vi "Find Virtual Sensor Readings NIARC 2016 Course (SubVI).vi"(8 "Lidar's Maximum Viewing Distance":dbl=5.6, 9 "Lidar Viewing Angle (degrees)":dbl=240.0, 10 "Number of Lidar Measurements":dbl=683.0, 11 "Position":cluster{"X":dbl, "Y":dbl, "Angle":dbl}) -> (1 "Angle":dbl[](array[numeric]), 2 "Magnitude":dbl[](array[numeric]))   [LabVIEW 2015]
panel:
  out "Polar Plot":picture
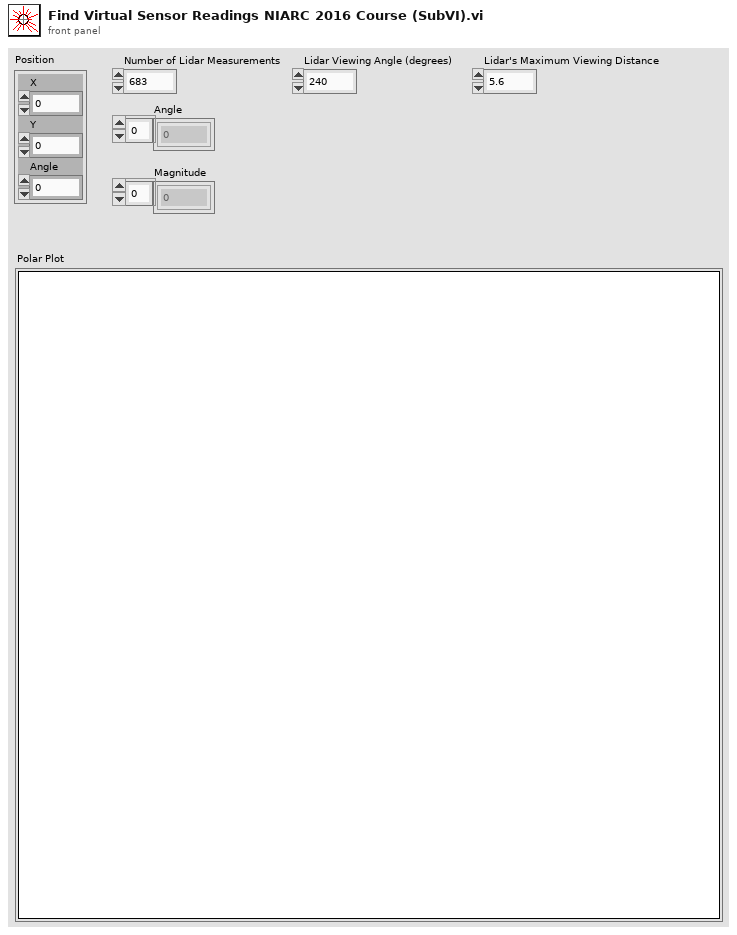
[diagram p1: front panel]
types:
  T1 = typedef "LVBoundsTypeDef.ctl" = cluster{"Width":u32, "Height":u32}
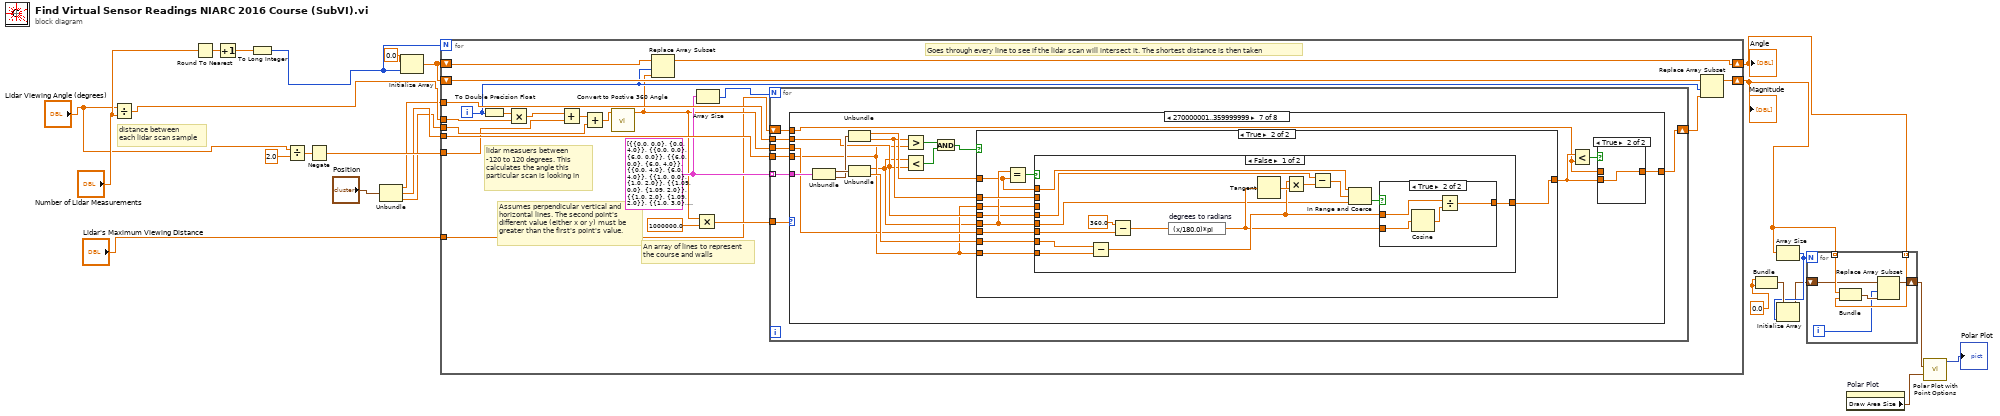
[diagram p0: block diagram]
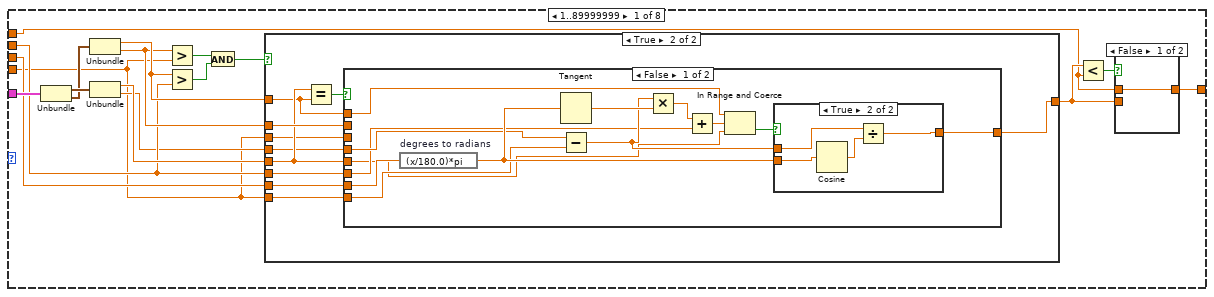
[diagram p2: hidden frame]
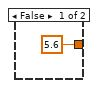
[diagram p4: hidden frame]
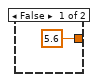
[diagram p5: hidden frame]
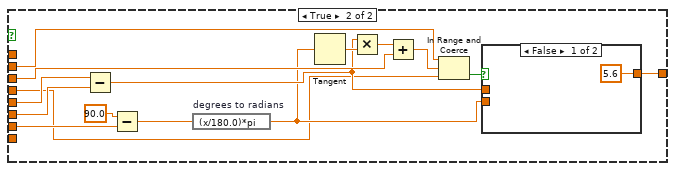
[diagram p6: hidden frame]
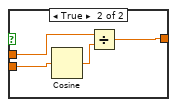
[diagram p7: hidden frame]
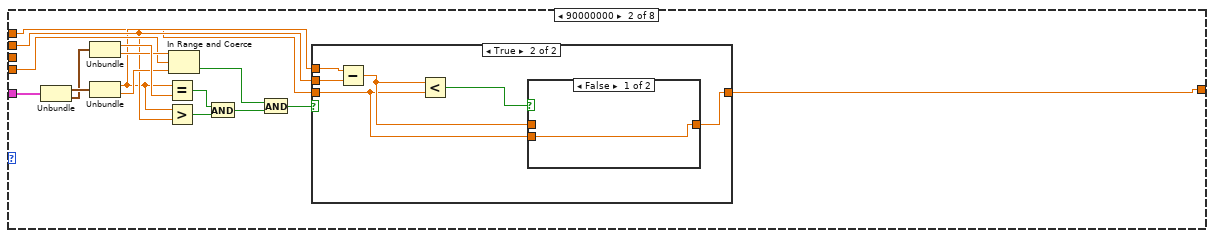
[diagram p8: hidden frame]
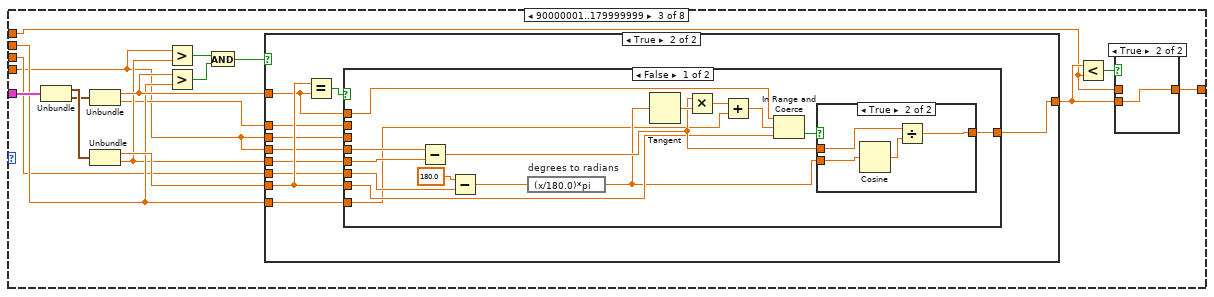
[diagram p11: hidden frame]
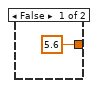
[diagram p13: hidden frame]
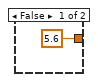
[diagram p14: hidden frame]
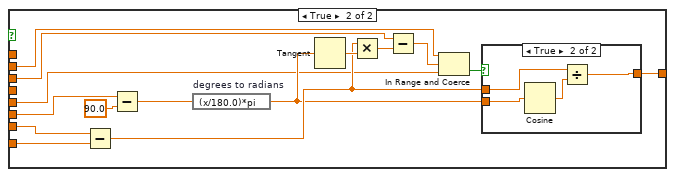
[diagram p15: hidden frame]
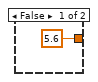
[diagram p16: hidden frame]
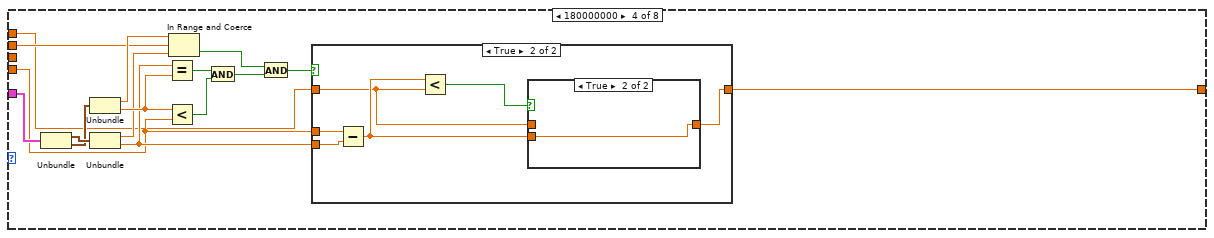
[diagram p17: hidden frame]
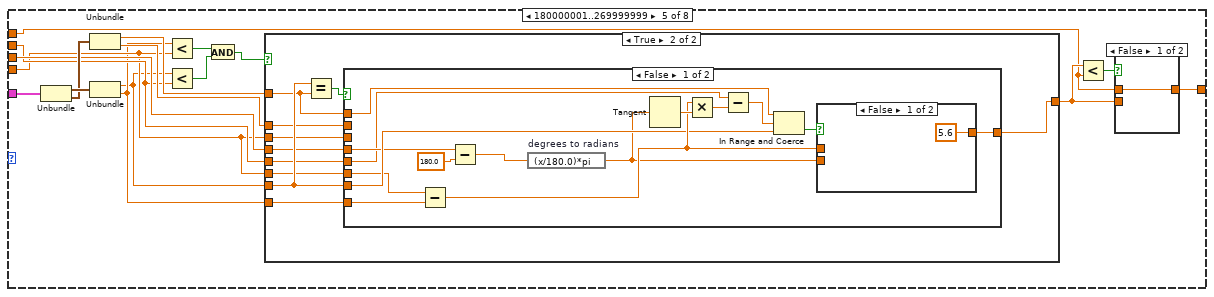
[diagram p20: hidden frame]
diagram:
  w4 = 0.0
  # "distance between\neach lidar scan sample"
  n1 = Divide(x="Lidar Viewing Angle (degrees)", y="Number of Lidar Measurements") -> (x/y=w22:dbl)
  n2 = Round To Nearest(number="Number of Lidar Measurements") -> (nearest integer value=w25:dbl)
  n3 = Increment(x=w25) -> (x+1=w24:dbl)
  n4 = To Long Integer(number=w24) -> (32bit integer=w23:i32)
  n5 = Divide(x="Lidar Viewing Angle (degrees)", y=2.0) -> (x/y=w19:dbl)
  n6 = Negate(x=w19) -> (-x=w16:dbl)
  n7 = Unbundle("Position") -> ("X"=w12:dbl, "Y"=w11:dbl, "Angle"=w10:dbl)
  n8 = Initialize Array(0.0 ("element"), w23) -> (w14:dbl[])
  n9 = for {
    N: w23 -> [_]
    tunnel: w10 -> [w40]
    tunnel: w12 -> [w45]
    tunnel: w11 -> [w44]
    tunnel: w22 -> [w43]
    shift-right: [w36] -> w7
    shift-left: w14 -> [w37]
    shift-right: [w28] -> w6
    shift-left: w14 -> [w30]
    tunnel: "Lidar's Maximum Viewing Distance" -> [w27]
    tunnel: w16 -> [w26]
    i -> [w31]
    w35 = cluster{cluster{dbl, dbl}, cluster{dbl, dbl}}[] [{{0.0, 0.0}, {0.0, 4.0}}, {{0.0, 0.0}, {6.0, 0.0}}, {{6.0, 0.0}, {6.0, 4.0}}, {{0.0, 4.0}, {6.0, 4.0}}, {{1.0, 0.0}, {1.0, 2.0}}, {{1.09, 0.0}, {1.09, 2.0}}, {{1.0, 2.0}, {1.09, 2.0}}, {{1.0, 3.0}, {1.0, 4.0}}, {{1.09, 3.0}, {1.09, 4.0}}, {{1.0, 3.0}, {1.09, 3.0}}, {{1.5, 3.88}, {1.5, 4.0}}, {{4.0, 3.88}, {4.0, 4.0}}, {{1.5, 3.88}, {4.0, 3.88}}, {{1.25, 0.0}, {1.25, 0.12}}, {{2.25, 0.0}, {2.25, 0.12}}, {{1.25, 0.12}, {2.25, 0.12}}, {{3.5, 0.0}, {3.5, 2.09}}, {{3.59, 0.0}, {3.59, 2.0}}, {{3.5, 2.09}, {4.5, 2.09}}, {{4.5, 2.0}, {4.5, 2.09}}, {{3.59, 2.0}, {4.5, 2.0}}, {{3.8, 0.0}, {3.8, 0.12}}, {{5.8, 0.0}, {5.8, 0.12}}, {{3.8, 0.12}, {5.8, 0.12}}]
    # "Assumes perpendicular vertical and\nhorizontal lines. The second point's\ndifferent value (either x or y) must be\ngreater than the first's point's value."
    # "Goes through every line to see if the lidar scan will intersect it. The shortest distance is then taken"
    # "An array of lines to represent\nthe course and walls"
    # "lidar measuers between\n-120 to 120 degrees. This\ncalculates the angle this \nparticular scan is looking in"
    n10 = To Double Precision Float(number=w31) -> (double precision float=w42:dbl)
    n11 = Multiply(x=w42, y=w43) -> (x*y=w41:dbl)
    n12 = Add(x=w41, y=w26) -> (x+y=w39:dbl)
    n13 = Add(x=w39, y=w40) -> (x+y=w32:dbl)
    n14 = call "Convert to Postive 360 Angle.vi"("Angle in"=w32) -> ("Angle out"=w29:dbl)  [unwired: 10 in]
    n15 = Replace Array Subset(array=w30, new element=w29, index=w31) -> (w28:dbl[])
    n16 = Multiply(x=w29, y=1000000.0) -> (x*y=w33:dbl)
    n17 = Array Size(array=w35) -> (size(s)=w46:i32)
    n18 = for {
      N: w46 -> [_]
      tunnel: w35 -> [w53] mode=indexing
      tunnel: w44 -> [w52]
      tunnel: w45 -> [w51]
      shift-right: [w49] -> w38
      shift-left: w27 -> [w50]
      tunnel: w29 -> [w48]
      tunnel: w33 -> [w47]
      n19 = case shown="270000001..359999999" w47 {
        tunnel: w53 -> [w68 w130 w155 w221 w249 w316 w343 w422]
        tunnel: w52 -> [w54 w126 w147 w220 w245 w313 w339 w409]
        tunnel: w51 -> [w61 w125 w153 w219 w247 w312 w340 w416]
        tunnel: w50 -> [w56 w123 w148 w218 w246 w314 w341 w408]
        tunnel: [w58 w122 w149 w217 w242 w315 w338 w407] -> w49
        tunnel: w48 -> [w60 _ w152 _ w248 _ w342 _]
        frame 1..89999999 {
          n20 = Unbundle(w68) -> (w70:cluster{dbl, dbl}, w69:cluster{dbl, dbl})
          n21 = Unbundle(w69) -> (w63:dbl, w62:dbl)
          n22 = Unbundle(w70) -> (w64:dbl, w55:dbl)
          n23 = Greater?(x=w62, y=w54) -> (0:w67:bool)
          n24 = Greater?(x=w63, y=w61) -> (0:w66:bool)
          n25 = And(x=w67, y=w66) -> (x .and. y?=w65:bool)
          n26 = case shown="True" w65 {
            tunnel: [5.6 w77] -> w57
            tunnel: w64 -> [_ w81]
            tunnel: w63 -> [_ w74]
            tunnel: w62 -> [_ w82]
            tunnel: w61 -> [_ w80]
            tunnel: w60 -> [_ w79]
            tunnel: w54 -> [_ w78]
            tunnel: w55 -> [_ w76]
            tunnel: w54 -> [_ w75]
            frame False {
            }
            frame True {
              n27 = Equal?(x=w81, y=w74) -> (x = y?=w83:bool)
              n28 = case shown="False" w83 {
                tunnel: w82 -> [_ w105]
                tunnel: w81 -> [w84 w116]
                tunnel: w80 -> [w89 w115]
                tunnel: w79 -> [w90 w114]
                tunnel: w78 -> [_ w109]
                tunnel: [w88 w106] -> w77
                tunnel: w76 -> [w92 w104]
                tunnel: w75 -> [w91 _]
                tunnel: w74 -> [w87 _]
                frame False {
                  n29 = expression code="(x/180.0)*pi" "degrees to radians"(w90) -> (w93:dbl)
                  n30 = Tangent(1:w93) -> (0:w96:dbl)
                  n31 = Subtract(x=w92, y=w91) -> (x-y=w94:dbl)
                  n32 = Multiply(x=w94, y=w96) -> (x*y=w95:dbl)
                  n33 = Add(x=w95, y=w89) -> (x+y=w86:dbl)
                  n34 = In Range and Coerce(upper limit=w87, x=w86, lower limit=w84) -> (In Range?=w85:bool)  [unwired: 1 out]
                  n35 = case shown="True" w85 {
                    tunnel: w94 -> [_ w101]
                    tunnel: w93 -> [_ w99]
                    tunnel: [5.6 w98] -> w88
                    frame False {
                    }
                    frame True {
                      n36 = Cosine(x=w99) -> (cos(x)=w100:dbl)
                      n37 = Divide(x=w101, y=w100) -> (x/y=w98:dbl)
                    }
                  }
                }
                frame True {
                  n38 = Subtract(x=w116, y=w115) -> (x-y=w108:dbl)
                  n39 = Subtract(x=90.0, y=w114) -> (x-y=w112:dbl)
                  n40 = expression code="(x/180.0)*pi" "degrees to radians"(w112) -> (w107:dbl)
                  n41 = Tangent(1:w107) -> (0:w111:dbl)
                  n42 = Multiply(x=w108, y=w111) -> (x*y=w110:dbl)
                  n43 = Add(x=w110, y=w109) -> (x+y=w103:dbl)
                  n44 = In Range and Coerce(upper limit=w105, x=w103, lower limit=w104) -> (In Range?=w102:bool)  [unwired: 1 out]
                  n45 = case shown="False" w102 {
                    tunnel: w108 -> [_ w121]
                    tunnel: w107 -> [_ w119]
                    tunnel: [5.6 w118] -> w106
                    frame False {
                    }
                    frame True {
                      n46 = Cosine(x=w119) -> (cos(x)=w120:dbl)
                      n47 = Divide(x=w121, y=w120) -> (x/y=w118:dbl)
                    }
                  }
                }
              }
            }
          }
          n48 = Less?(x=w57, y=w56) -> (x < y?=w59:bool)
          n49 = case shown="False" w59 {
            tunnel: [w71 w72] -> w58
            tunnel: w57 -> [_ w72]
            tunnel: w56 -> [w71 _]
            frame False {
            }
            frame True {
            }
          }
        }
        frame 90000000 {
          n50 = Unbundle(w130) -> (w137:cluster{dbl, dbl}, w136:cluster{dbl, dbl})
          n51 = Unbundle(w136) -> (w129:dbl, w127:dbl)
          n52 = Unbundle(w137) -> (w124:dbl, w128:dbl)
          n53 = Equal?(x=w124, y=w129) -> (x = y?=w134:bool)
          n54 = Greater?(x=w124, y=w125) -> (0:w135:bool)
          n55 = In Range and Coerce(upper limit=w127, x=w126, lower limit=w128) -> (In Range?=w132:bool)  [unwired: 1 out]
          n56 = And(x=w134, y=w135) -> (x .and. y?=w133:bool)
          n57 = And(x=w132, y=w133) -> (x .and. y?=w131:bool)
          n58 = case shown="True" w131 {
            tunnel: [w138 w143] -> w122
            tunnel: w125 -> [_ w141]
            tunnel: w124 -> [_ w140]
            tunnel: w123 -> [w138 w139]
            frame False {
            }
            frame True {
              n59 = Subtract(x=w140, y=w141) -> (x-y=w142:dbl)
              n60 = Less?(x=w142, y=w139) -> (x < y?=w144:bool)
              n61 = case shown="False" w144 {
                tunnel: [w145 w146] -> w143
                tunnel: w142 -> [_ w146]
                tunnel: w139 -> [w145 _]
                frame False {
                }
                frame True {
                }
              }
            }
          }
        }
        frame 90000001..179999999 {
          n62 = Unbundle(w155) -> (w163:cluster{dbl, dbl}, w162:cluster{dbl, dbl})
          n63 = Unbundle(w162) -> (w154:dbl, w150:dbl)
          n64 = Unbundle(w163) -> (w158:dbl, w151:dbl)
          n65 = Greater?(x=w147, y=w151) -> (0:w161:bool)
          n66 = Greater?(x=w154, y=w153) -> (0:w160:bool)
          n67 = And(x=w161, y=w160) -> (x .and. y?=w159:bool)
          n68 = case shown="True" w159 {
            tunnel: [5.6 w174] -> w156
            tunnel: w158 -> [_ w175]
            tunnel: w154 -> [_ w172]
            tunnel: w151 -> [_ w173]
            tunnel: w153 -> [_ w171]
            tunnel: w152 -> [_ w170]
            tunnel: w147 -> [_ w169]
            tunnel: w150 -> [_ w168]
            tunnel: w147 -> [_ w167]
            frame False {
            }
            frame True {
              n69 = Equal?(x=w175, y=w172) -> (x = y?=w176:bool)
              n70 = case shown="False" w176 {
                tunnel: w175 -> [w184 w211]
                tunnel: [w188 w206] -> w174
                tunnel: w173 -> [w183 w205]
                tunnel: w172 -> [w187 _]
                tunnel: w171 -> [w177 w203]
                tunnel: w170 -> [w179 w201]
                tunnel: w169 -> [_ w198]
                tunnel: w168 -> [_ w197]
                tunnel: w167 -> [w182 _]
                frame False {
                  n71 = Subtract(x=w182, y=w183) -> (x-y=w189:dbl)
                  n72 = Subtract(x=180.0, y=w179) -> (x-y=w181:dbl)
                  n73 = expression code="(x/180.0)*pi" "degrees to radians"(w181) -> (w178:dbl)
                  n74 = Tangent(1:w178) -> (0:w191:dbl)
                  n75 = Multiply(x=w189, y=w191) -> (x*y=w190:dbl)
                  n76 = Add(x=w190, y=w177) -> (x+y=w186:dbl)
                  n77 = In Range and Coerce(upper limit=w187, x=w186, lower limit=w184) -> (In Range?=w185:bool)  [unwired: 1 out]
                  n78 = case shown="True" w185 {
                    tunnel: w189 -> [_ w196]
                    tunnel: w178 -> [_ w194]
                    tunnel: [5.6 w193] -> w188
                    frame False {
                    }
                    frame True {
                      n79 = Cosine(x=w194) -> (cos(x)=w195:dbl)
                      n80 = Divide(x=w196, y=w195) -> (x/y=w193:dbl)
                    }
                  }
                }
                frame True {
                  n81 = Subtract(x=w211, y=w203) -> (x-y=w208:dbl)
                  n82 = Subtract(x=w201, y=90.0 ("x")) -> (x-y=w210:dbl)
                  n83 = expression code="(x/180.0)*pi" "degrees to radians"(w210) -> (w207:dbl)
                  n84 = Tangent(1:w207) -> (0:w209:dbl)
                  n85 = Multiply(x=w208, y=w209) -> (x*y=w199:dbl)
                  n86 = Subtract(x=w198, y=w199) -> (x-y=w200:dbl)
                  n87 = In Range and Coerce(upper limit=w197, x=w200, lower limit=w205) -> (In Range?=w204:bool)  [unwired: 1 out]
                  n88 = case shown="True" w204 {
                    tunnel: w208 -> [_ w216]
                    tunnel: w207 -> [_ w214]
                    tunnel: [5.6 w213] -> w206
                    frame False {
                    }
                    frame True {
                      n89 = Cosine(x=w214) -> (cos(x)=w215:dbl)
                      n90 = Divide(x=w216, y=w215) -> (x/y=w213:dbl)
                    }
                  }
                }
              }
            }
          }
          n91 = Less?(x=w156, y=w148) -> (x < y?=w157:bool)
          n92 = case shown="True" w157 {
            tunnel: [w164 w165] -> w149
            tunnel: w156 -> [_ w165]
            tunnel: w148 -> [w164 _]
            frame False {
            }
            frame True {
            }
          }
        }
        frame 180000000 {
          n93 = Unbundle(w221) -> (w232:cluster{dbl, dbl}, w231:cluster{dbl, dbl})
          n94 = Unbundle(w231) -> (w226:dbl, w230:dbl)
          n95 = Unbundle(w232) -> (w227:dbl, w222:dbl)
          n96 = Equal?(x=w222, y=w230) -> (x = y?=w228:bool)
          n97 = Less?(x=w230, y=w220) -> (x < y?=w229:bool)
          n98 = In Range and Coerce(upper limit=w226, x=w219, lower limit=w227) -> (In Range?=w224:bool)  [unwired: 1 out]
          n99 = And(x=w228, y=w229) -> (x .and. y?=w225:bool)
          n100 = And(x=w224, y=w225) -> (x .and. y?=w223:bool)
          n101 = case shown="True" w223 {
            tunnel: w222 -> [_ w234]
            tunnel: w220 -> [_ w235]
            tunnel: w218 -> [w233 w236]
            tunnel: [w233 w238] -> w217
            frame False {
            }
            frame True {
              n102 = Subtract(x=w235, y=w234) -> (x-y=w237:dbl)
              n103 = Less?(x=w237, y=w236) -> (x < y?=w239:bool)
              n104 = case shown="True" w239 {
                tunnel: [w240 w241] -> w238
                tunnel: w237 -> [_ w241]
                tunnel: w236 -> [w240 _]
                frame False {
                }
                frame True {
                }
              }
            }
          }
        }
        frame 180000001..269999999 {
          n105 = Unbundle(w249) -> (w258:cluster{dbl, dbl}, w257:cluster{dbl, dbl})
          n106 = Unbundle(w257) -> (w251:dbl, w250:dbl)
          n107 = Unbundle(w258) -> (w243:dbl, w244:dbl)
          n108 = Less?(x=w244, y=w245) -> (x < y?=w256:bool)
          n109 = Less?(x=w243, y=w247) -> (x < y?=w255:bool)
          n110 = And(x=w256, y=w255) -> (x .and. y?=w254:bool)
          n111 = case shown="True" w254 {
            tunnel: [5.6 w269] -> w252
            tunnel: w243 -> [_ w270]
            tunnel: w251 -> [_ w267]
            tunnel: w244 -> [_ w268]
            tunnel: w247 -> [_ w266]
            tunnel: w248 -> [_ w265]
            tunnel: w245 -> [_ w264]
            tunnel: w250 -> [_ w263]
            tunnel: w245 -> [_ w262]
            frame False {
            }
            frame True {
              n112 = Equal?(x=w270, y=w267) -> (x = y?=w271:bool)
              n113 = case shown="False" w271 {
                tunnel: w270 -> [w280 w293]
                tunnel: [w284 w302] -> w269
                tunnel: w268 -> [w279 w301]
                tunnel: w267 -> [w283 _]
                tunnel: w266 -> [w272 w292]
                tunnel: w265 -> [w275 w294]
                tunnel: w264 -> [_ w297]
                tunnel: w263 -> [_ w296]
                tunnel: w262 -> [w278 _]
                frame False {
                  n114 = Subtract(x=w278, y=w279) -> (x-y=w285:dbl)
                  n115 = Subtract(x=w275, y=180.0 ("x")) -> (x-y=w274:dbl)
                  n116 = expression code="(x/180.0)*pi" "degrees to radians"(w274) -> (w277:dbl)
                  n117 = Tangent(1:w277) -> (0:w286:dbl)
                  n118 = Multiply(x=w285, y=w286) -> (x*y=w273:dbl)
                  n119 = Subtract(x=w272, y=w273) -> (x-y=w282:dbl)
                  n120 = In Range and Coerce(upper limit=w283, x=w282, lower limit=w280) -> (In Range?=w281:bool)  [unwired: 1 out]
                  n121 = case shown="False" w281 {
                    tunnel: w285 -> [_ w291]
                    tunnel: w277 -> [_ w289]
                    tunnel: [5.6 w288] -> w284
                    frame False {
                    }
                    frame True {
                      n122 = Cosine(x=w289) -> (cos(x)=w290:dbl)
                      n123 = Divide(x=w291, y=w290) -> (x/y=w288:dbl)
                    }
                  }
                }
                frame True {
                  n124 = Subtract(x=w292, y=w293) -> (x-y=w304:dbl)
                  n125 = Subtract(x=270.0, y=w294) -> (x-y=w306:dbl)
                  n126 = expression code="(x/180.0)*pi" "degrees to radians"(w306) -> (w303:dbl)
                  n127 = Tangent(1:w303) -> (0:w305:dbl)
                  n128 = Multiply(x=w304, y=w305) -> (x*y=w298:dbl)
                  n129 = Subtract(x=w297, y=w298) -> (x-y=w299:dbl)
                  n130 = In Range and Coerce(upper limit=w296, x=w299, lower limit=w301) -> (In Range?=w300:bool)  [unwired: 1 out]
                  n131 = case shown="True" w300 {
                    tunnel: w304 -> [_ w311]
                    tunnel: w303 -> [_ w309]
                    tunnel: [5.6 w308] -> w302
                    frame False {
                    }
                    frame True {
                      n132 = Cosine(x=w309) -> (cos(x)=w310:dbl)
                      n133 = Divide(x=w311, y=w310) -> (x/y=w308:dbl)
                    }
                  }
                }
              }
            }
          }
          n134 = Less?(x=w252, y=w246) -> (x < y?=w253:bool)
          n135 = case shown="False" w253 {
            tunnel: [w259 w260] -> w242
            tunnel: w252 -> [_ w260]
            tunnel: w246 -> [w259 _]
            frame False {
            }
            frame True {
            }
          }
        }
        frame 270000000 {
          n136 = Unbundle(w316) -> (w327:cluster{dbl, dbl}, w326:cluster{dbl, dbl})
          n137 = Unbundle(w326) -> (w320:dbl, w318:dbl)
          n138 = Unbundle(w327) -> (w317:dbl, w319:dbl)
          n139 = Equal?(x=w317, y=w320) -> (x = y?=w324:bool)
          n140 = Less?(x=w317, y=w312) -> (x < y?=w325:bool)
          n141 = In Range and Coerce(upper limit=w318, x=w313, lower limit=w319) -> (In Range?=w322:bool)  [unwired: 1 out]
          n142 = And(x=w324, y=w325) -> (x .and. y?=w323:bool)
          n143 = And(x=w322, y=w323) -> (x .and. y?=w321:bool)
          n144 = case shown="True" w321 {
            tunnel: [w328 w333] -> w315
            tunnel: w312 -> [_ w331]
            tunnel: w317 -> [_ w330]
            tunnel: w314 -> [w328 w329]
            frame False {
            }
            frame True {
              n145 = Subtract(x=w331, y=w330) -> (x-y=w332:dbl)
              n146 = Less?(x=w332, y=w329) -> (x < y?=w334:bool)
              n147 = case shown="False" w334 {
                tunnel: [w335 w336] -> w333
                tunnel: w332 -> [_ w336]
                tunnel: w329 -> [w335 _]
                frame False {
                }
                frame True {
                }
              }
            }
          }
        }
        frame 270000001..359999999 {
          n148 = Unbundle(w343) -> (w353:cluster{dbl, dbl}, w352:cluster{dbl, dbl})
          n149 = Unbundle(w352) -> (w348:dbl, w347:dbl)
          n150 = Unbundle(w353) -> (w337:dbl, w344:dbl)
          n151 = Greater?(x=w347, y=w339) -> (0:w351:bool)
          n152 = Less?(x=w337, y=w340) -> (x < y?=w350:bool)
          n153 = And(x=w351, y=w350) -> (x .and. y?=w349:bool)
          n154 = case shown="True" w349 {
            tunnel: [5.6 w360] -> w345
            tunnel: w337 -> [_ w364]
            tunnel: w348 -> [_ w357]
            tunnel: w347 -> [_ w365]
            tunnel: w340 -> [_ w363]
            tunnel: w342 -> [_ w362]
            tunnel: w339 -> [_ w361]
            tunnel: w344 -> [_ w359]
            tunnel: w339 -> [_ w358]
            frame False {
            }
            frame True {
              n155 = Equal?(x=w364, y=w357) -> (x = y?=w366:bool)
              n156 = case shown="False" w366 {
                tunnel: w365 -> [_ w394]
                tunnel: w364 -> [w372 w390]
                tunnel: w363 -> [w369 w389]
                tunnel: w362 -> [w367 w387]
                tunnel: w361 -> [_ w398]
                tunnel: [w376 w395] -> w360
                tunnel: w359 -> [w378 w393]
                tunnel: w358 -> [w377 _]
                tunnel: w357 -> [w375 _]
                frame False {
                  n157 = Subtract(x=w378, y=w377) -> (x-y=w380:dbl)
                  n158 = Subtract(x=360.0 ("y"), y=w367) -> (x-y=w371:dbl)
                  n159 = expression code="(x/180.0)*pi" "degrees to radians"(w371) -> (w379:dbl)
                  n160 = Tangent(1:w379) -> (0:w381:dbl)
                  n161 = Multiply(x=w380, y=w381) -> (x*y=w370:dbl)
                  n162 = Subtract(x=w369, y=w370) -> (x-y=w374:dbl)
                  n163 = In Range and Coerce(upper limit=w375, x=w374, lower limit=w372) -> (In Range?=w373:bool)  [unwired: 1 out]
                  n164 = case shown="True" w373 {
                    tunnel: w380 -> [_ w386]
                    tunnel: w379 -> [_ w384]
                    tunnel: [5.6 w383] -> w376
                    frame False {
                    }
                    frame True {
                      n165 = Cosine(x=w384) -> (cos(x)=w385:dbl)
                      n166 = Divide(x=w386, y=w385) -> (x/y=w383:dbl)
                    }
                  }
                }
                frame True {
                  n167 = Subtract(x=w389, y=w390) -> (x-y=w397:dbl)
                  n168 = Subtract(x=w387, y=270.0 ("x")) -> (x-y=w401:dbl)
                  n169 = expression code="(x/180.0)*pi" "degrees to radians"(w401) -> (w396:dbl)
                  n170 = Tangent(1:w396) -> (0:w400:dbl)
                  n171 = Multiply(x=w397, y=w400) -> (x*y=w399:dbl)
                  n172 = Add(x=w399, y=w398) -> (x+y=w392:dbl)
                  n173 = In Range and Coerce(upper limit=w394, x=w392, lower limit=w393) -> (In Range?=w391:bool)  [unwired: 1 out]
                  n174 = case shown="True" w391 {
                    tunnel: w397 -> [_ w406]
                    tunnel: w396 -> [_ w404]
                    tunnel: [5.6 w403] -> w395
                    frame False {
                    }
                    frame True {
                      n175 = Cosine(x=w404) -> (cos(x)=w405:dbl)
                      n176 = Divide(x=w406, y=w405) -> (x/y=w403:dbl)
                    }
                  }
                }
              }
            }
          }
          n177 = Less?(x=w345, y=w341) -> (x < y?=w346:bool)
          n178 = case shown="True" w346 {
            tunnel: [w354 w355] -> w338
            tunnel: w345 -> [_ w355]
            tunnel: w341 -> [w354 _]
            frame False {
            }
            frame True {
            }
          }
        }
        frame 0, Default {
          n179 = Unbundle(w422) -> (w421:cluster{dbl, dbl}, w420:cluster{dbl, dbl})
          n180 = Unbundle(w420) -> (w414:dbl, w419:dbl)
          n181 = Unbundle(w421) -> (w415:dbl, w410:dbl)
          n182 = Equal?(x=w410, y=w419) -> (x = y?=w417:bool)
          n183 = Greater?(x=w419, y=w409) -> (0:w418:bool)
          n184 = In Range and Coerce(upper limit=w414, x=w416, lower limit=w415) -> (In Range?=w412:bool)  [unwired: 1 out]
          n185 = And(x=w417, y=w418) -> (x .and. y?=w413:bool)
          n186 = And(x=w412, y=w413) -> (x .and. y?=w411:bool)
          n187 = case shown="True" w411 {
            tunnel: w410 -> [_ w429]
            tunnel: w409 -> [_ w428]
            tunnel: w408 -> [w423 w424]
            tunnel: [w423 w426] -> w407
            frame False {
            }
            frame True {
              n188 = Subtract(x=w429, y=w428) -> (x-y=w425:dbl)
              n189 = Less?(x=w425, y=w424) -> (x < y?=w427:bool)
              n190 = case shown="False" w427 {
                tunnel: [w430 w431] -> w426
                tunnel: w425 -> [_ w431]
                tunnel: w424 -> [w430 _]
                frame False {
                }
                frame True {
                }
              }
            }
          }
        }
      }
    }
    n191 = Replace Array Subset(array=w37, new element=w38, index=w31) -> (w36:dbl[])
  }
  "Angle" <- w6
  "Magnitude" <- w7
  n192 = Bundle(w4, w4) -> (w5:cluster{dbl, dbl})  [unwired: 1 in]
  n193 = Array Size(array=w7) -> (size(s)=w3:i32)
  n194 = Initialize Array(w5, w3) -> (w2:cluster{dbl, dbl}[])
  n195 = for {
    N: w3 -> [_]
    tunnel: w7 -> [w437] mode=indexing
    tunnel: w6 -> [w436] mode=indexing
    shift-right: [w432] -> w1
    shift-left: w2 -> [w433]
    i -> [w434]
    n196 = Bundle("element"=w437, "element"=w436) -> (w435:cluster{"element":dbl, "element":dbl})  [unwired: 1 in]
    n197 = Replace Array Subset(array=w433, new element=w435, index=w434) -> (w432:cluster{dbl, dbl}[])
  }
  n198 = property on="Polar Plot" class="Pict"() -> ("Draw Area Size"=w8:T1)  [unwired: 2 in, 2 out]
  n199 = call <vilib>:"Polar Plot with Point Options.vi"("data array [mag, phase (deg)]"=w1, "dimensions (w,h)"=w8) -> ("new picture"=→"Polar Plot":picture)  [unwired: 13 in]
